vi "Set Filter Parameters.vi"(5 "noise":i32, 6 "smooth":i32, 7 "accept":sgl, 9 "range":i32, 10 "sensitivity":sgl, 11 "width":i32) -> (3 "function return":u32)   [LabVIEW 2018, in "AndorSDK.lvlib"]
doc: "EXPNETTYPE unsigned int WINAPI SetFilterParameters(int width, float sensitivity, int range, float accept, int smooth, int noise);"
uses:
  AndorSDK.lvlib
  ATMCD32D.dll
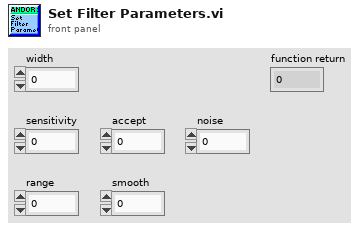
[diagram p1: front panel]
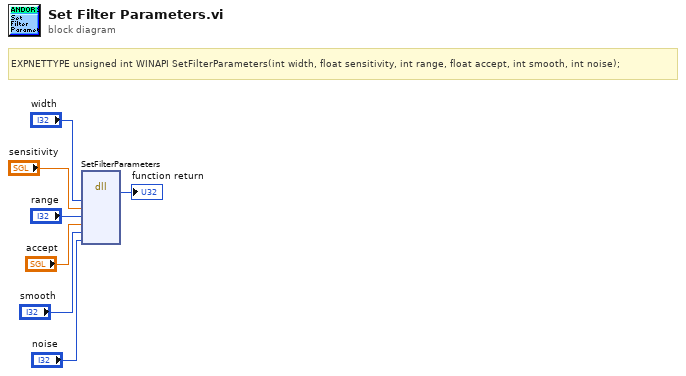
[diagram p0: block diagram]
diagram:
  # "EXPNETTYPE unsigned int WINAPI SetFilterParameters(int width, float sensitivity, int range, float accept, int smooth, int noise);"
  n1 = dll-call lib="PTH2babs E\nPersönliches02 - Arbeit03-HiwijobsLabviewCodelibANDOR\tAndor SDK\nATMCD32D.*" fn="SetFilterParameters"("width"="width", "sensitivity"="sensitivity", "range"="range", "accept"="accept", "smooth"="smooth", "noise"="noise") -> (→"function return":u32)  [unwired: 9 in, 2 out]
